vi "Initialize.vi"(8 "error in":errorcluster, 11 "Pump Calibration Config in":T1={"Settings"={"Cycle Period"=500.0, "Ismatech"={"VISA resource name"="", "Simulated?"=TRUE, "Pump Number"=1.0, "Reverse?"=FALSE}, "Masterflex"={"VISA resource name"="", "Simulated?"=TRUE, "Pump Number"=1.0, "Reverse?"=FALSE}, "Bronkhorst M13 Settings"={"VISA resource name"="", "Simulated?"=TRUE, "Smoothing Steps"=1}, "PID 2 Parameters"={"Input Device"=enum."Default", "Output Device"=enum."Default"}, "Tacmina Settings"={"Analog DAQ Task"="", "Digital DAQ Task"=""}, "KNF SIMDOS Settings"={"VISA resource name"="", "Simulated?"=TRUE}, "VICI M50 Settings"={"VISA resource name"="", "Pump ID"="", "Pump Head Vol"=0.0, "Reverse?"=FALSE, "Simulated?"=TRUE}, "FLOM Settings"={"VISA resource name"="", "Simulated?"=TRUE, "Pump Number"=0.0}, "Calibration Limits"={"Minimum (ml/min)"=0.0, "Maximum (ml/min)"=0.0, "Steps"=0.0}, "SSI PR Settings"={"VISA resource name"="", "Simulated?"=FALSE}, "Ismatech 4308 Settings"={"VISA resource name"="", "Pump Number"=1, "Channel Number"=0, "Simulated?"=TRUE, "Reverse?"=FALSE}, "Bronkhorst M14 Settings"={"VISA resource name"="", "Simulated?"=FALSE, "Smoothing Steps"=1}}, "Flowmeter Output"=0.0, "Density"=0.0, "FL Temp"=0.0, "Speed %"=0.0, "File Refnum"=refnum, "Pump On?"=enum."Not Initialized"} {"Settings"."Bronkhorst M14 Settings"."Smoothing Steps" min=1 step=1; "Settings"."Ismatech 4308 Settings"."Channel Number" min=0 max=3; "Settings"."Ismatech 4308 Settings"."Pump Number" min=1; "Settings"."Bronkhorst M13 Settings"."Smoothing Steps" min=1 step=1; "Settings"."Masterflex"."Pump Number" min=1.0 max=20.0 step=1.0; "Settings"."Ismatech"."Pump Number" min=1.0 max=20.0 step=1.0}) -> (0 "error out":errorcluster, 3 "Pump Calibration Config Out":T1={"Settings"={"Cycle Period"=500.0, "Ismatech"={"VISA resource name"="", "Simulated?"=TRUE, "Pump Number"=1.0, "Reverse?"=FALSE}, "Masterflex"={"VISA resource name"="", "Simulated?"=TRUE, "Pump Number"=1.0, "Reverse?"=FALSE}, "Bronkhorst M13 Settings"={"VISA resource name"="", "Simulated?"=TRUE, "Smoothing Steps"=1}, "PID 2 Parameters"={"Input Device"=enum."Default", "Output Device"=enum."Default"}, "Tacmina Settings"={"Analog DAQ Task"="", "Digital DAQ Task"=""}, "KNF SIMDOS Settings"={"VISA resource name"="", "Simulated?"=TRUE}, "VICI M50 Settings"={"VISA resource name"="", "Pump ID"="", "Pump Head Vol"=0.0, "Reverse?"=FALSE, "Simulated?"=TRUE}, "FLOM Settings"={"VISA resource name"="", "Simulated?"=TRUE, "Pump Number"=0.0}, "Calibration Limits"={"Minimum (ml/min)"=0.0, "Maximum (ml/min)"=0.0, "Steps"=0.0}, "SSI PR Settings"={"VISA resource name"="", "Simulated?"=FALSE}, "Ismatech 4308 Settings"={"VISA resource name"="", "Pump Number"=1, "Channel Number"=0, "Simulated?"=TRUE, "Reverse?"=FALSE}, "Bronkhorst M14 Settings"={"VISA resource name"="", "Simulated?"=FALSE, "Smoothing Steps"=1}}, "Flowmeter Output"=0.0, "Density"=0.0, "FL Temp"=0.0, "Speed %"=0.0, "File Refnum"=refnum, "Pump On?"=enum."Not Initialized"} {"Settings"."Bronkhorst M14 Settings"."Smoothing Steps" min=1 step=1; "Settings"."Ismatech 4308 Settings"."Channel Number" min=0 max=3; "Settings"."Ismatech 4308 Settings"."Pump Number" min=1; "Settings"."Bronkhorst M13 Settings"."Smoothing Steps" min=1 step=1; "Settings"."Masterflex"."Pump Number" min=1.0 max=20.0 step=1.0; "Settings"."Ismatech"."Pump Number" min=1.0 max=20.0 step=1.0})   [LabVIEW 2018, in "Calibration.lvlib" / "Engine.lvlib"]
uses:
  Engine.lvlib
  Pump Calibration Config.ctl
  Pfizer Timed Seq/Software/Ismatec ISM 831C/Controls/Ismatech ISM831C Settings Cluster.ctl
  Pfizer Timed Seq/Software/Masterflex 7550-30/Controls/Settings Cluster.ctl
  Pfizer Timed Seq/Software/Bronkhorst M13 Flow Meter/Settings Cluster.ctl
  Pfizer Timed Seq/Software/Measure Instrument/PID Input Enum.ctl
  Pfizer Timed Seq/Software/Measure Instrument/PID 2 Output Enum.ctl
  Pfizer Timed Seq/Software/Tacmina QI/Tacmina QI DAQ Setting.ctl
  Pfizer Timed Seq/Software/KNF Pump/Settings Cluster plus SIMDOS.ctl
  Pfizer Timed Seq/Software/VICI M50 Party Mode/Settings Cluster.ctl
  Pfizer Timed Seq/Software/FLOM Pump/Settings Cluster.ctl
  Pfizer Timed Seq/Software/SSI PR Class/SSI PR or LD Settings Cluster.ctl
  Pfizer Timed Seq/Software/Ismatec 78001/Ismatec 4083.ctl
  Pfizer Timed Seq/Software/Bronkhorst M14 Flow Meter/Settings Cluster.ctl
  Pfizer Timed Seq/Software/Bronkhorst M13 Flow Meter/Bronkhorst M13 Flow Meter.lvlib
  Pfizer Timed Seq/Software/Bronkhorst M14 Flow Meter/Bronkhorst M14 Flow Meter.lvlib
  Pfizer Timed Seq/Software/Ismatec ISM 831C/Ismatec ISM 831C.lvlib
  Pfizer Timed Seq/Software/Masterflex 7550-30/Masterflex 7550-30.lvlib
  Pfizer Timed Seq/Software/VICI M50 Party Mode/VICI M6 M50 Party Mode.lvlib
  Pfizer Timed Seq/Software/Tacmina QI/Tacmina QI.lvlib
  Pfizer Timed Seq/Software/KNF Pump/KNF SIMDOS.lvlib
  Pfizer Timed Seq/Software/FLOM Pump/FLOM Pump.lvlib
  Pfizer Timed Seq/Software/Ismatec 78001/Ismatec 4308.lvlib
  Pfizer Timed Seq/Software/Calibration VIs/Calibration.lvlib
  Pfizer Timed Seq/Software/SSI PR Class/SSI PR or LD Pump.lvlib
panel:
  # "Output Instruments"
  # "Input Instruments"
  # "Output Instruments"
  # "Input Instruments"
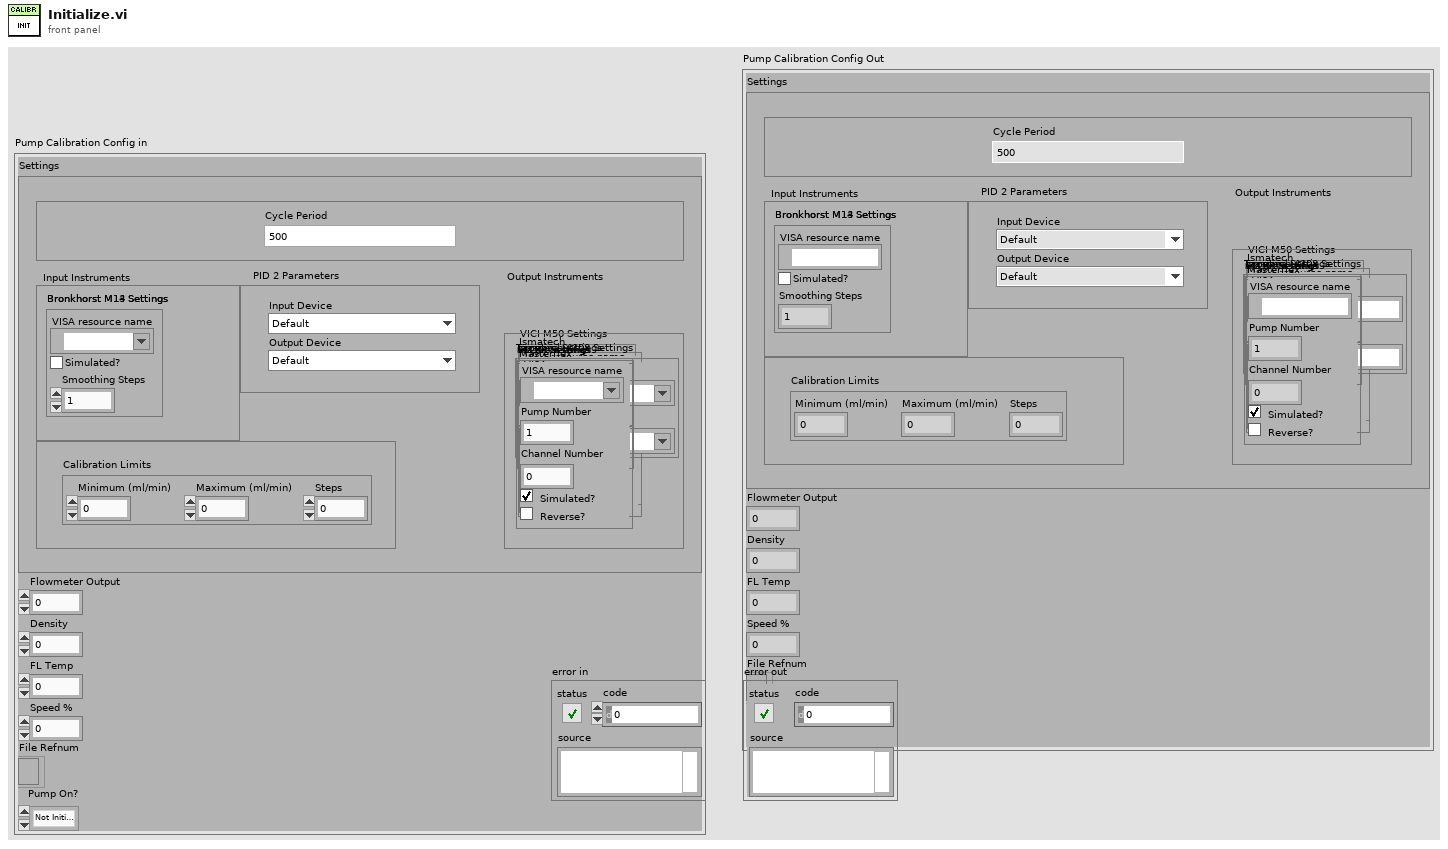
[diagram p1: front panel]
types:
  T1 = typedef "Calibration.lvlib/Pump Calibration Config.ctl" = cluster{"Settings":cluster{"Cycle Period":dbl, "Ismatech":T2, "Masterflex":T3, "Bronkhorst M13 Settings":T4, "PID 2 Parameters":cluster{"Input Device":T5, "Output Device":T6}, "Tacmina Settings":T7, "KNF SIMDOS Settings":T8, "VICI M50 Settings":T9, "FLOM Settings":T10, "Calibration Limits":cluster{"Minimum (ml/min)":dbl, "Maximum (ml/min)":dbl, "Steps":dbl}, "SSI PR Settings":T11, "Ismatech 4308 Settings":T12, "Bronkhorst M14 Settings":T13}, "Flowmeter Output":dbl, "Density":dbl, "FL Temp":dbl, "Speed %":dbl, "File Refnum":refnum<file>, "Pump On?":enum16{"Off", "On", "Not Initialized"}}
  T2 = typedef "Ismatec ISM 831C.lvlib/Ismatech ISM831C Settings Cluster.ctl" = cluster{"VISA resource name":refnum<visa-resource-name>, "Simulated?":bool, "Pump Number":dbl, "Reverse?":bool}
  T3 = typedef "Masterflex 7550-30.lvlib/Settings Cluster.ctl" = cluster{"VISA resource name":refnum<visa-resource-name>, "Simulated?":bool, "Pump Number":dbl, "Reverse?":bool}
  T4 = typedef "Bronkhorst M13 Flow Meter.lvlib/Settings Cluster.ctl" = cluster{"VISA resource name":refnum<visa-resource-name>, "Simulated?":bool, "Smoothing Steps":i32}
  T5 = typedef "PID Input Enum.ctl" = enum16{"Default", "Bronkhorst M13", "Bronkhorst M14", "Scale Rate of Change"}
  T6 = typedef "PID 2 Output Enum.ctl" = enum16{"Default", "Ismatec ISM 4308", "Ismatec ISM 831C", "Masterflex 7550-30", "VICI M6", "VICI M50", "Tacmina QI", "KNF SIMDOS", "ASIA Type C", "FLOM UI-22-11", "SSI PR/LD", "SSI P40", "Masterflex 75211-70"}
  T7 = typedef "Tacmina QI.lvlib/Tacmina QI DAQ Setting.ctl" = cluster{"Analog DAQ Task":refnum<k21>, "Digital DAQ Task":refnum<k21>}
  T8 = typedef "KNF SIMDOS.lvlib/Settings Cluster plus SIMDOS.ctl" = cluster{"VISA resource name":refnum<visa-resource-name>, "Simulated?":bool}
  T9 = typedef "VICI M6 M50 Party Mode.lvlib/Settings Cluster.ctl" = cluster{"VISA resource name":refnum<visa-resource-name>, "Pump ID":string, "Pump Head Vol":dbl, "Reverse?":bool, "Simulated?":bool}
  T10 = typedef "FLOM Pump.lvlib/Settings Cluster.ctl" = cluster{"VISA resource name":refnum<visa-resource-name>, "Simulated?":bool, "Pump Number":dbl}
  T11 = typedef "SSI PR or LD Pump.lvlib/SSI PR or LD Settings Cluster.ctl" = cluster{"VISA resource name":refnum<visa-resource-name>, "Simulated?":bool}
  T12 = typedef "Ismatec 4308.lvlib/Ismatec 4083.ctl" = cluster{"VISA resource name":refnum<visa-resource-name>, "Pump Number":i16, "Channel Number":i16, "Simulated?":bool, "Reverse?":bool}
  T13 = typedef "Bronkhorst M14 Flow Meter.lvlib/Settings Cluster.ctl" = cluster{"VISA resource name":refnum<visa-resource-name>, "Simulated?":bool, "Smoothing Steps":i32}
  T14 = cluster{"Cycle Period":dbl, "Ismatech":T2, "Masterflex":T3, "Bronkhorst M13 Settings":T4, "PID 2 Parameters":cluster{"Input Device":T5, "Output Device":T6}, "Tacmina Settings":T7, "KNF SIMDOS Settings":T8, "VICI M50 Settings":T9, "FLOM Settings":T10, "Calibration Limits":cluster{"Minimum (ml/min)":dbl, "Maximum (ml/min)":dbl, "Steps":dbl}, "SSI PR Settings":T11, "Ismatech 4308 Settings":T12, "Bronkhorst M14 Settings":T13}
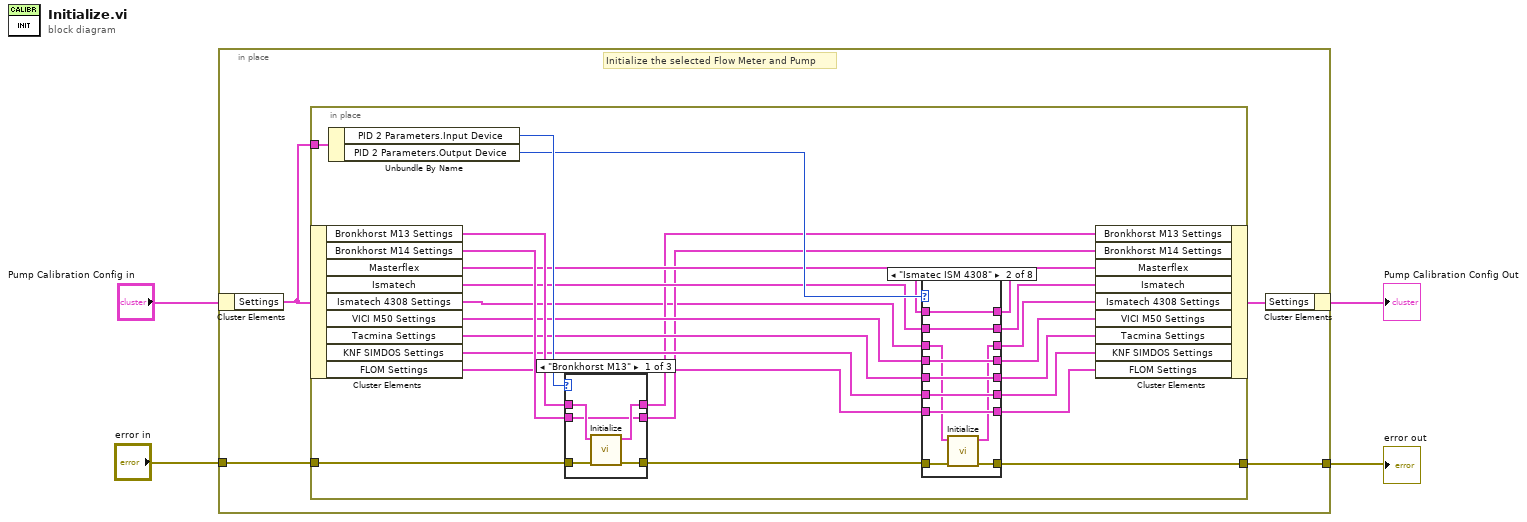
[diagram p0: block diagram]
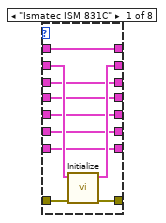
[diagram p2: hidden frame]
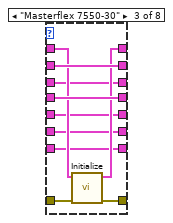
[diagram p3: hidden frame]
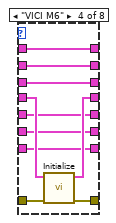
[diagram p4: hidden frame]
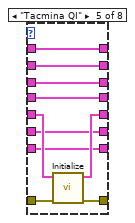
[diagram p5: hidden frame]
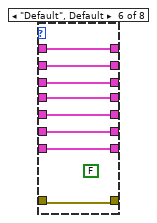
[diagram p6: hidden frame]
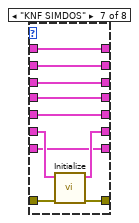
[diagram p7: hidden frame]
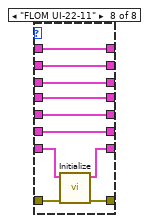
[diagram p8: hidden frame]
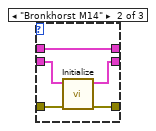
[diagram p9: hidden frame]
diagram:
  n1 = in-place {
    in-place-border: "error in" -> [w8]
    in-place-border: [w7] -> w1
    # "Initialize the selected Flow Meter and Pump"
    n2 = in-place-cluster #1("Pump Calibration Config in") -> ("Settings"=w6:T14)
    n3 = in-place {
      in-place-border: w8 -> [w32]
      in-place-border: w6 -> [w28]
      in-place-border: [w27] -> w7
      n4 = in-place-cluster #2(w6) -> ("Bronkhorst M13 Settings"=w26:T4, "Bronkhorst M14 Settings"=w25:T13, "Masterflex"=w24:T3, "Ismatech"=w23:T2, "Ismatech 4308 Settings"=w10:T12, "VICI M50 Settings"=w22:T9, "Tacmina Settings"=w21:T7, "KNF SIMDOS Settings"=w20:T8, "FLOM Settings"=w19:T10)
      n5 = Unbundle By Name(w28) -> ("PID 2 Parameters.Input Device"=w31:T5, "PID 2 Parameters.Output Device"=w30:T6)
      n6 = case shown="\"Bronkhorst M13\"" w31 {
        tunnel: w26 -> [w115 w118 w123]
        tunnel: w32 -> [w114 w120 w122]
        tunnel: [w113 w119 w122] -> w29
        tunnel: [w112 w118 w123] -> w18
        tunnel: w25 -> [w111 w117 w121]
        tunnel: [w111 w116 w121] -> w17
        frame "Bronkhorst M13" {
          n7 = call "Initialize.vi"("error in (no error)"=w114, "Bronkhorst Settings in"=w115) -> ("error out"=w113:errorcluster, "Bronkhorst Settings out"=w112:T4)  [unwired: 7 in, 1 out]
        }
        frame "Bronkhorst M14" {
          n8 = call "Initialize.vi"("error in (no error)"=w120, "Bronkhorst Settings in"=w117) -> ("error out"=w119:errorcluster, "Bronkhorst Settings out"=w116:T13)  [unwired: 7 in, 1 out]
        }
        frame "Default", Default {
        }
      }
      n9 = case shown="\"Ismatec ISM 4308\"" w30 {
        tunnel: w24 -> [w39 w52 w60 w67 w79 w90 w100 w110]
        tunnel: [w39 w52 w59 w67 w79 w90 w100 w110] -> w16
        tunnel: w29 -> [w42 w46 w57 w69 w81 w88 w96 w105]
        tunnel: [w38 w43 w58 w70 w82 w88 w95 w104] -> w27
        tunnel: w23 -> [w41 w51 w62 w68 w80 w89 w99 w109]
        tunnel: [w40 w51 w62 w68 w80 w89 w99 w109] -> w15
        tunnel: w22 -> [w37 w50 w61 w72 w78 w86 w98 w108]
        tunnel: [w37 w50 w61 w71 w78 w86 w98 w108] -> w14
        tunnel: w21 -> [w36 w49 w56 w66 w77 w87 w97 w107]
        tunnel: [w36 w49 w56 w66 w76 w87 w97 w107] -> w13
        tunnel: w20 -> [w35 w48 w55 w65 w75 w85 w93 w106]
        tunnel: [w35 w48 w55 w65 w75 w85 w94 w106] -> w12
        tunnel: w19 -> [w34 w47 w54 w64 w74 w84 w92 w102]
        tunnel: [w34 w47 w54 w64 w74 w84 w92 w103] -> w11
        tunnel: w10 -> [w33 w45 w53 w63 w73 w83 w91 w101]
        tunnel: [w33 w44 w53 w63 w73 w83 w91 w101] -> w9
        frame "Ismatec ISM 831C" {
          n10 = call "Initialize.vi"("error in (no error)"=w42, "Ismatech Settings"=w41) -> ("error out"=w38:errorcluster, "Ismatech Settings"=w40:T2)  [unwired: 6 in, 2 out]
        }
        frame "Ismatec ISM 4308" {
          n11 = call "Initialize.vi"("error in (no error)"=w46, "Ismatech 3 Channel Settings In"=w45) -> ("error out"=w43:errorcluster, "Ismatech 3 Channel Settings Out"=w44:T12)  [unwired: 6 in, 2 out]
        }
        frame "Masterflex 7550-30" {
          n12 = call "Initialize.vi"("error in (no error)"=w57, "Masterflex Settings in"=w60) -> ("error out"=w58:errorcluster, "Masterflex Settings out"=w59:T3)  [unwired: 6 in, 2 out]
        }
        frame "VICI M6" {
          n13 = call "Initialize.vi"("error in (no error)"=w69, "VICI Settings"=w72) -> ("error out"=w70:errorcluster, "VICI Settings"=w71:T9)  [unwired: 6 in, 2 out]
        }
        frame "Tacmina QI" {
          n14 = call "Initialize.vi"("error in"=w81, "Tacmina Settings in"=w77) -> ("error out"=w82:errorcluster, "Tacmina Settings out"=w76:T7)  [unwired: 7 in, 1 out]
        }
        frame "Default", Default {
          (unwired) FALSE ("Initialized")
        }
        frame "KNF SIMDOS" {
          n15 = call "Initialize.vi"("error in (no error)"=w96, "KNF Settings In"=w93) -> ("error IO"=w95:errorcluster, "KNF Settings Out"=w94:T8)  [unwired: 6 in, 2 out]
        }
        frame "FLOM UI-22-11" {
          n16 = call "Initialize.vi"("error in (no error)"=w105, "FLOM Settings in"=w102) -> ("error out"=w104:errorcluster, "FLOM Settings out"=w103:T10)  [unwired: 6 in, 2 out]
        }
      }
      n17 = in-place-cluster #2("Bronkhorst M13 Settings"=w18, "Bronkhorst M14 Settings"=w17, "Masterflex"=w16, "Ismatech"=w15, "Ismatech 4308 Settings"=w9, "VICI M50 Settings"=w14, "Tacmina Settings"=w13, "KNF SIMDOS Settings"=w12, "FLOM Settings"=w11) -> (w5:T14)
    }
    n18 = in-place-cluster #1("Settings"=w5) -> (→"Pump Calibration Config Out":T1)
  }
  "error out" <- w1
